vi "pr2b1.vi"() -> ()   [LabVIEW 2013]
uses:
  <vilib>/Platform/TimedLoop/XDataNode/timing_clust.ctl
  <vilib>/Platform/TimedLoop/XDataNode/nitl_modes.ctl
  <vilib>/Platform/TimedLoop/XDataNode/wakeup.ctl
  <vilib>/DAQmx/write.llb/DAQmx Write (Counter Frequency 1Chan 1Samp).vi
  <vilib>/DAQmx/read.llb/DAQmx Read (Counter DBL 1Chan 1Samp).vi
  <vilib>/DAQmx/write.llb/DAQmx Write (Digital Bool 1Line 1Point).vi
  <vilib>/DAQmx/create/channels.llb/DAQmx Create Channel (CI-Position-Angular Encoder).vi
  <vilib>/DAQmx/create/channels.llb/DAQmx Create Channel (DO-Digital Output).vi
  <vilib>/DAQmx/create/channels.llb/DAQmx Create Channel (CO-Pulse Generation-Frequency).vi
  <vilib>/DAQmx/configure/timing.llb/DAQmx Timing (Implicit).vi
  <vilib>/DAQmx/miscellaneous.llb/DAQmx Fill In Error Info.vi
  <vilib>/platform/TimedLoop/XDataNode/XDataNode.xnode
  <vilib>/Platform/TimedLoop/XDataNode/XDNodeRunTimeDep.lvlib
panel:
  in  "Señal a generar":enum16{"Chirp", "Archivo"}(ring)=enum."Archivo"
  out "offset":dbl
  in  "Rango Frec para chrip":cluster{"start freq":dbl, "end freq":dbl}={"start freq"=0.5, "end freq"=2.0} {"end freq" format="%0.2f"; "start freq" format="%0.2f"}
  in  "Puntos a generar-chirp":i32=100
  in  "amplitude":dbl=0.1 format="%0.2f"
  in  "Zona muerta":dbl=0.2
  out "Y max":dbl format="%0.2f"
  out "Señales Normalizadas":waveform(dbl)[](graph)
  out "RPM":waveform(dbl)(graph)
  in  "Numero de ciclos de \nPWM por periodo de muestreo (N)":dbl=20.0
  in  "Counter (s)":tag="Dev1/ctr0"
  in  "Periodo de muestreo (seg)":dbl=0.05
  out "Señal de entrada (DC)":waveform(dbl)(graph)
  out "Error":errorcluster
  in  "Salida para DIR":tag="Dev1/port0/line0"
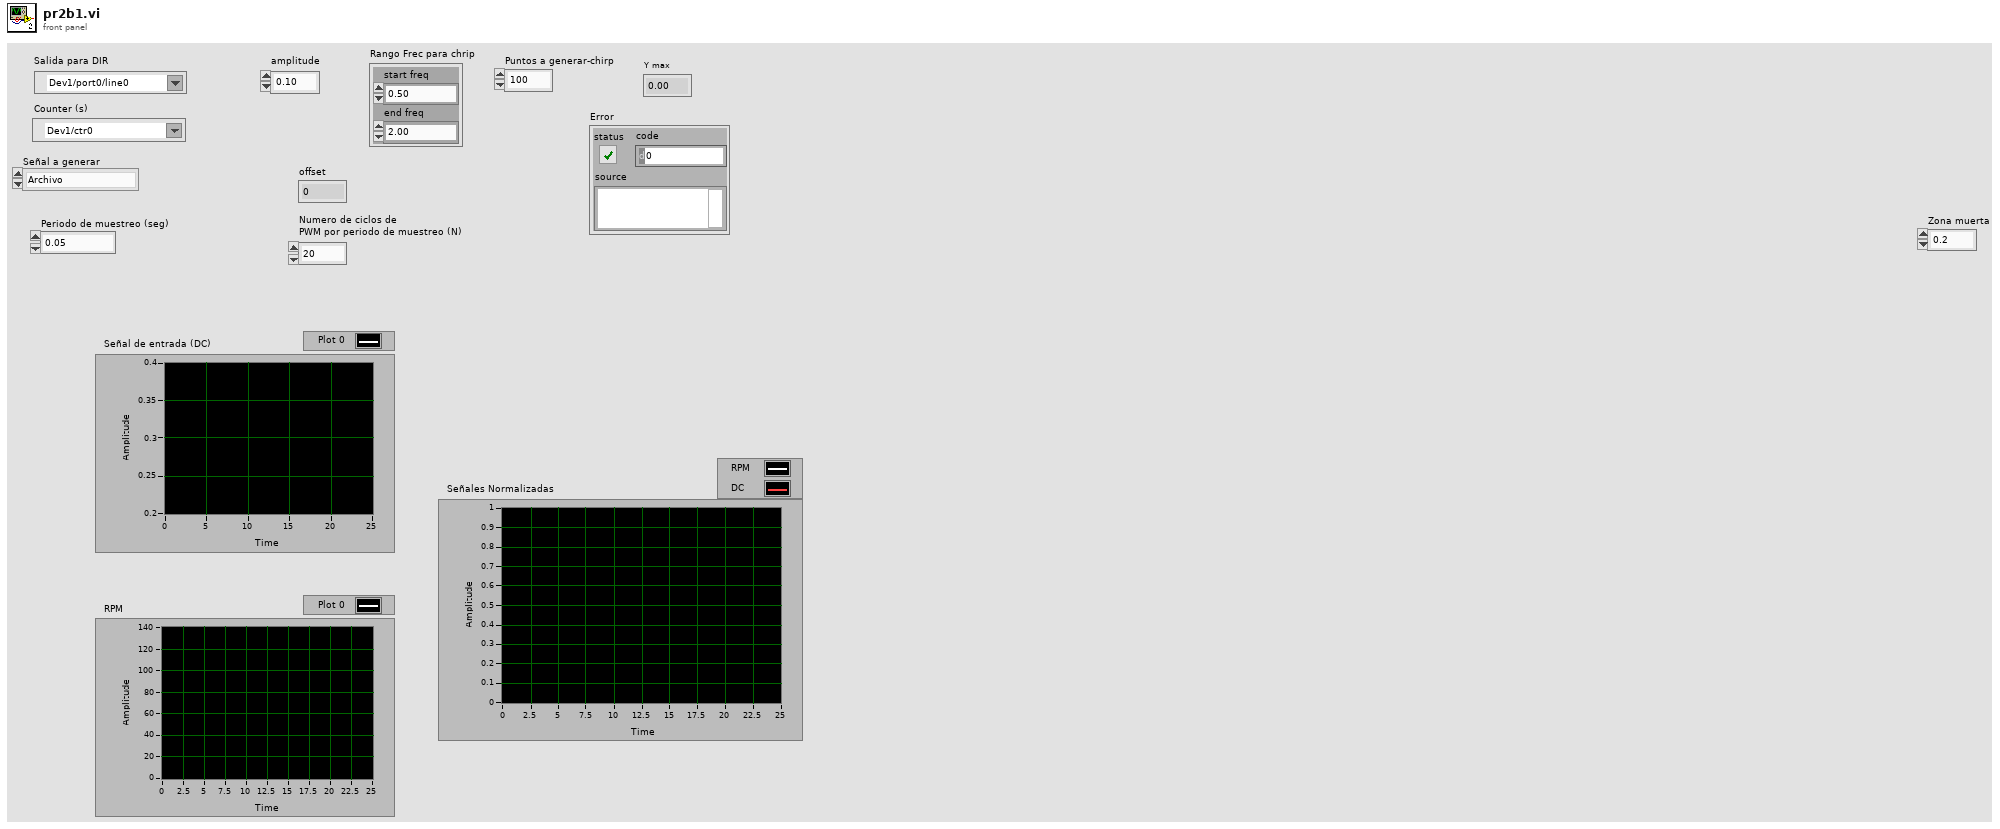
[diagram p1: front panel]
types:
  T1 = typedef "XDNodeRunTimeDep.lvlib/timing_clust.ctl" = cluster{"Expected End [f-1]":u64, "Actual End [f-1]":u64, "Finished Late? [f-1]":bool, "Expected End [i-1]":u64, "Actual End [i-1]":u64, "Finished Late? [i-1]":bool, "Expected Start [i]":u64, "Actual Start [i]":u64, "Expected Start [f]":u64, "Actual Start [f]":u64, "Source Name":string, "Structure Name":string, "Period":i64, "Deadline":i64, "Offset":i64, "Start":i64, "Priority":i32, "Timeout":i32, "Mode":T2, "Wakeup Reason":T3, "Error":errorcluster, "Source Type":string, "Secondary Source Type":string, "Global End Time":u64, "Global Start Time":u64, "Frame Duration":u64, "Iteration Duration":u64, "Assigned CPU":i32, "I/O Scan Engine Mode":u32}
  T2 = typedef "XDNodeRunTimeDep.lvlib/nitl_modes.ctl" = enum32{"No Change", "Process missed periods, maintain original phase", "Discard missed periods, maintain original phase", "Process missed periods, ignore original phase", "Discard missed periods, ignore original phase"}
  T3 = typedef "XDNodeRunTimeDep.lvlib/wakeup.ctl" = enum32{"Normal", "Aborted", "Asynchronous wakeup", "Timing source error", "Timed loop error", "Timeout"}
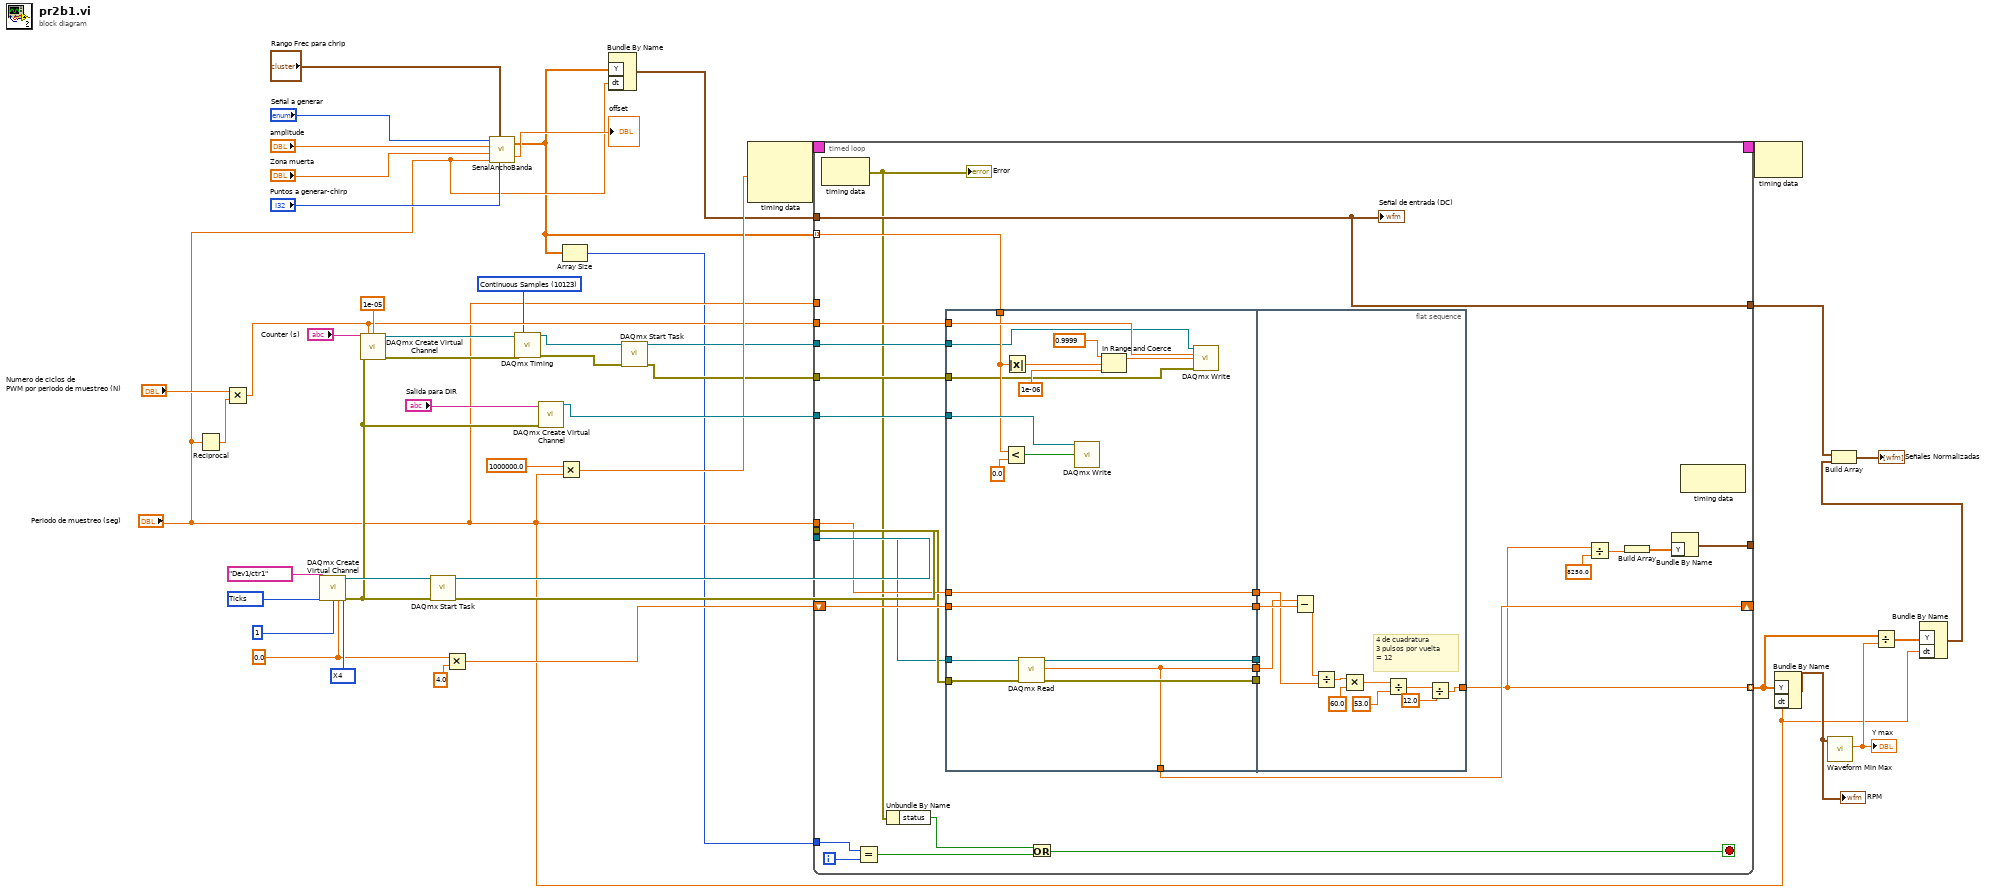
[diagram p0: block diagram]
diagram:
  w18 = 10123 items=["Finite Samples"=10178, "Continuous Samples"=10123, "Hardware Timed Single Point"=12522] ("sample mode")
  w41 = 10092 items=["X1"=10090, "X2"=10091, "X4"=10092, "Two Pulse Counting"=10313] ("decoding type")
  w36 = 0.0 ("initial angle")
  w43 = 10304 items=["Degrees"=10146, "Radians"=10273, "Ticks"=10304, "From Custom Scale"=10065] ("units")
  n1 = Reciprocal(x="Periodo de muestreo (seg)") -> (1/x=w25:dbl)
  n2 = Multiply(x="Numero de ciclos de \nPWM por periodo de muestreo (N)", y=w25) -> (x*y=w26:dbl)
  n3 = call-poly <vilib>:"DAQmx Create Virtual Channel.vi"("counter"=tag "Dev1/ctr1", "decoding type"=w41, "units"=w43, "pulses per revolution"=u32 1, "initial angle"=w36) -> ("task out"=w40:refnum<k21>, "error out"=w28:errorcluster)  [unwired: 9 in]
  n4 = call-poly <vilib>:"DAQmx Create Virtual Channel.vi"("frequency"=w26, "duty cycle"=1e-05, "counter"="Counter (s)", "error in"=w28) -> ("task out"=w24:refnum<k21>, "error out"=w21:errorcluster)  [unwired: 10 in]
  n5 = call <vilib>:"DAQmx Start Task.vi"("task/channels in"=w40, "error in"=w28) -> ("task out"=w39:refnum<k21>, "error out"=w38:errorcluster)  [unwired: 12 in]
  n6 = Multiply(x=w36, y=4.0) -> (x*y=w27:dbl)
  n7 = call "SenalAnchoBanda.vi"("Puntos a generar-chirp"="Puntos a generar-chirp", "Rango Frec para chrip"="Rango Frec para chrip", "Tm"="Periodo de muestreo (seg)", "Zona muerta"="Zona muerta", "amplitude"="amplitude", "Señal a generar"="Señal a generar") -> ("offset"=→"offset":dbl, "Señal"=w3:dbl[])
  n8 = call-poly <vilib>:"DAQmx Timing.vi"("task/channels in"=w24, "sample mode"=w18, "error in"=w21) -> ("task out"=w23:refnum<k21>, "error out"=w20:errorcluster)  [unwired: 11 in]
  n9 = call-poly <vilib>:"DAQmx Create Virtual Channel.vi"("lines"="Salida para DIR", "error in"=w28) -> ("task out"=w33:refnum<k21>)  [unwired: 12 in, 1 out]
  n10 = Multiply(x=1000000.0, y="Periodo de muestreo (seg)") -> (x*y=w32:dbl)
  n11 = Array Size(array=w3) -> (size(s)=w2:i32)
  n12 = Bundle By Name("Y"=w3, "dt"="Periodo de muestreo (seg)") -> (w4:waveform(dbl))  [unwired: 1 in]
  n13 = call <vilib>:"DAQmx Start Task.vi"("task/channels in"=w23, "error in"=w20) -> ("task out"=w22:refnum<k21>, "error out"=w19:errorcluster)  [unwired: 12 in]
  n14 = node-c288(w32) -> (w46:T1)  [unwired: 2 in]
  n15 = timed-loop {
    timing: w46 -> [_]
    timing-out: [_] -> w45
    shift-right: [w64] -> _
    shift-left: w27 -> [w73]
    tunnel: w39 -> [w66]
    tunnel: w38 -> [w67]
    tunnel: "Periodo de muestreo (seg)" -> [w72]
    tunnel: w3 -> [w60] mode=indexing
    tunnel: "Periodo de muestreo (seg)" -> [_]
    tunnel: w33 -> [w69]
    tunnel: w4 -> [w57]
    tunnel: w26 -> [w61]
    tunnel: w22 -> [w59]
    tunnel: w19 -> [w58]
    tunnel: [w55] -> w15 mode=indexing
    tunnel: [w57] -> w17
    tunnel: w2 -> [w56]
    tunnel: [w51] -> _
    i -> [w62]
    stop <- w47 stop-if-true
    n16 = node-c288() -> (w50:errorcluster)  [unwired: 1 in]
    "Error" <- w50
    n17 = Equal?(x=w56, y=w62) -> (x = y?=w49:bool)
    n18 = Unbundle By Name(w50) -> ("status"=w48:bool)
    n19 = flat-sequence {
      tunnel: w72 -> [w90]
      tunnel: w73 -> [w91]
      tunnel: [w91] -> w71
      tunnel: [w90] -> w70
      tunnel: w69 -> [w85]
      tunnel: [w82] -> w68
      tunnel: w67 -> [w81]
      tunnel: w66 -> [w80]
      tunnel: [w79] -> w65
      tunnel: [w78] -> w64
      tunnel: [w78] -> w63
      tunnel: w61 -> [w77]
      tunnel: w60 -> [w76]
      tunnel: w59 -> [w75]
      tunnel: w58 -> [w74]
      tunnel: [w93] -> w55
      tunnel: w71 -> [w102]
      tunnel: w70 -> [w96]
      tunnel: w68 -> [_]
      tunnel: w65 -> [_]
      tunnel: w63 -> [w95]
      frame #0 {
        n20 = Less?(x=w76, y=0.0) -> (x < y?=w83:bool)
        n21 = Absolute Value(x=w76) -> (abs(x)=w87:dbl)
        n22 = call-poly <vilib>:"DAQmx Read.vi"("task/channels in"=w80, "error in"=w81) -> ("task out"=w79:refnum<k21>, "data"=w78:dbl, "error out"=w82:errorcluster)  [unwired: 11 in]
        n23 = call-poly <vilib>:"DAQmx Write.vi"("task/channels in"=w85, "data"=w83) -> ()  [unwired: 11 in, 3 out]
        n24 = In Range and Coerce(upper limit=0.9999, x=w87, lower limit=1e-06) -> (coerced(x)=w86:dbl)  [unwired: 1 out]
        n25 = call-poly <vilib>:"DAQmx Write.vi"("task/channels in"=w75, "frequency"=w77, "duty cycle"=w86, "error in"=w74) -> ()  [unwired: 9 in, 3 out]
      }
      frame #1 {
        # "4 de cuadratura\n3 pulsos por vuelta\n= 12"
        n26 = Subtract(x=w95, y=w102) -> (x-y=w101:dbl)
        n27 = Divide(x=w101, y=w96) -> (x/y=w100:dbl)
        n28 = Multiply(x=w100, y=60.0) -> (x*y=w98:dbl)
        n29 = Divide(x=w98, y=53.0) -> (x/y=w94:dbl)
        n30 = Divide(x=w94, y=12.0) -> (x/y=w93:dbl)
      }
    }
    n31 = Or(x=w48, y=w49) -> (x .or. y?=w47:bool)
    n32 = Divide(x=w55, y=8250.0) -> (x/y=w53:dbl)
    n33 = Build Array(w53) -> (w52:dbl[])
    n34 = Bundle By Name("Y"=w52) -> (w51:waveform(dbl))  [unwired: 1 in]
    n35 = node-c288() -> ()  [unwired: 1 in, 1 out]
    "Señal de entrada (DC)" <- w57
  }
  n36 = node-c288(w45) -> ()  [unwired: 1 out]
  n37 = Bundle By Name("Y"=w15, "dt"="Periodo de muestreo (seg)") -> (w11:waveform(dbl))  [unwired: 1 in]
  "RPM" <- w11
  n38 = call <vilib>:"Waveform Min Max.vi"("waveform in"=w11) -> ("Y max"=w14:dbl)  [unwired: 5 in, 5 out]
  "Y max" <- w14
  n39 = Divide(x=w15, y=w14) -> (x/y=w13:dbl[])
  n40 = Bundle By Name("Y"=w13, "dt"="Periodo de muestreo (seg)") -> (w12:waveform(dbl))  [unwired: 1 in]
  n41 = Build Array(w17, w12) -> (→"Señales Normalizadas":waveform(dbl)[])
